vi "VisionGlobals.vi"() -> ()   [LabVIEW 2020]
panel:
  in  "TargetID":i32
  in  "YOffset":dbl
  in  "XOffset":dbl
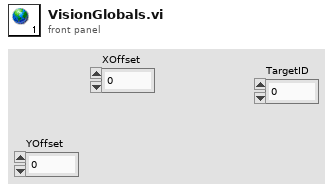
[diagram p1: front panel]
diagram:
